vi "RSZVB Get Generator Frequency Conversion.vi"(0 "VISA session":refnum<visa-resource-name>, 5 "Channel (1)":i32=1, 7 "Port (1)":i32=1, 9 "Generator Number (1)":i32=1, 11 "error in (no error)":errorcluster {"code" format="%.0x"}) -> (2 "Denominator":i32, 3 "Offset":dbl format="%^.3e", 4 "dup VISA session":refnum<visa-resource-name>, 6 "State":bool, 8 "Numerator":i32, 14 "Sweep Type":i32, 15 "error out":errorcluster {"code" format="%.0x"})   [LabVIEW 2011]
doc: "This VI returns an external generator frequency for frequency-converting measurements. The external generator frequency is either a range (for frequency sweeps) or a CW frequency (for power, time and CW Mode sweeps).\n\nNote(s):\n\n(1) This VI is available only on R&S ZVA instrument.\n\nRemote-control command(s):\nSOURce<Ch>:FREQuency<Pt>:CONVersion:ARBitrary:EFRequency<Gen>?"
uses:
  _utility/RSZVB Global Data.vi
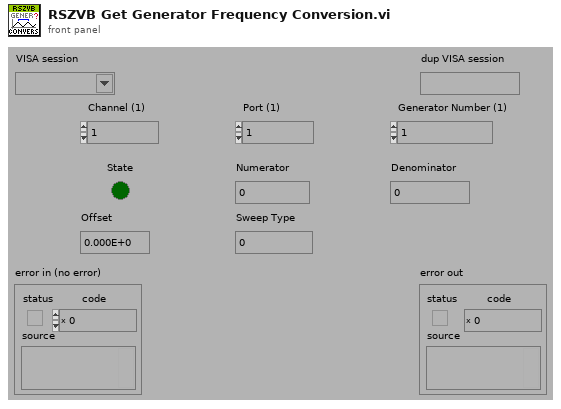
[diagram p1: front panel]
types:
  T1 = cluster{"Error Checking (T: On)":bool, "Installed Options":string[], "Data Valid?":bool, "Ports":i32, "Model":string[], "Option Checking (T: On)":bool}[]
  T2 = cluster{"Error Checking (T: On)":bool, "Installed Options":string[], "Data Valid?":bool, "Ports":i32, "Model":string[], "Option Checking (T: On)":bool}
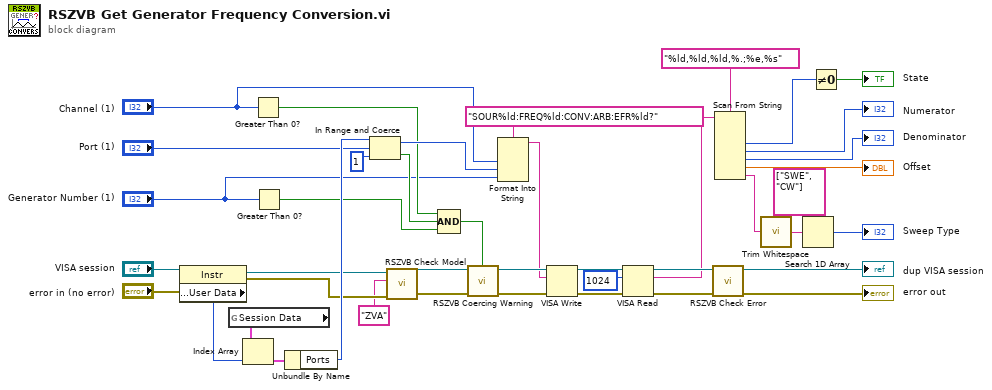
[diagram p0: block diagram]
diagram:
  n1 = property class="Instr"(reference="VISA session", error in="error in (no error)") -> (reference out=w23:refnum<visa-resource-name>, error out=w22:errorcluster, "General Settings:User Data"=w41:u32)
  n2 = global read "RSZVB Global Data.vi" "Session Data"() -> (w40:T1)
  n3 = Index Array(array=w40, index=w41) -> (element=w39:T2)
  n4 = Greater Than 0?(x="Channel (1)") -> (x > 0?=w8:bool)
  n5 = Greater Than 0?(x="Generator Number (1)") -> (x > 0?=w10:bool)
  n6 = Unbundle By Name(w39) -> ("Ports"=w37:i32)
  n7 = In Range and Coerce(upper limit=w37, x="Port (1)", lower limit=1) -> (coerced(x)=w11:i32, In Range?=w9:bool)
  n8 = call "RSZVB Check Model.vi"("error in (no error)"=w22, "Model"="ZVA" ("Options"), "VISA session"=w23) -> ("error out"=w25:errorcluster, "dup VISA session"=w24:refnum<visa-resource-name>)  [unwired: 7 in]
  n9 = Compound Arithmetic op=AND(w8, w9, w10) -> (w38:bool)
  n10 = call "RSZVB Coercing Warning.vi"("In Range?"=w38, "error in (no error)"=w25, "VISA session"=w24) -> ("error out"=w36:errorcluster, "dup VISA session"=w35:refnum<visa-resource-name>)  [unwired: 7 in]
  n11 = Format Into String(format string="SOUR%ld:FREQ%ld:CONV:ARB:EFR%ld?", "Channel (1)", w11, "Generator Number (1)") -> (resulting string=w19:string)  [unwired: 2 in, 1 out]
  n12 = VISA Write(VISA resource name=w35, write buffer=w19, error in (no error)=w36) -> (VISA resource name out=w29:refnum<visa-resource-name>, error out=w30:errorcluster)  [unwired: 1 out]
  n13 = VISA Read(VISA resource name=w29, byte count=u32 1024 ("byte count (0)"), error in (no error)=w30) -> (VISA resource name out=w33:refnum<visa-resource-name>, read buffer=w26:string, error out=w32:errorcluster)  [unwired: 1 out]
  n14 = call "RSZVB Check Error.vi"("error in (no error)"=w32, "VISA session"=w33) -> ("error out"=→"error out":errorcluster, "dup VISA session"=→"dup VISA session":refnum<visa-resource-name>)  [unwired: 8 in]
  n15 = Scan From String(format string="%ld,%ld,%ld,%.;%e,%s", input string=w26) -> (output 1=w1:i32, output 2=→"Numerator":i32, output 3=→"Denominator":i32, output 4=→"Offset":dbl, output 5=w5:string)  [unwired: 7 in, 3 out]
  n16 = call <vilib>:"Trim Whitespace.vi"("string"=w5) -> ("trimmed string"=w27:string)  [unwired: 1 in]
  n17 = Search 1D Array(1D array=string[] ["SWE", "CW"] ("array 2"), element=w27) -> (index of element=→"Sweep Type":i32)  [unwired: 1 in]
  n18 = Not Equal To 0?(x=w1) -> (x != 0?=→"State":bool)
